vi "s-6 metin belgesindeki datayı dışarı aktaran, okunmasını sağlayan program 2018 19.vi"() -> ()   [LabVIEW 2014]
panel:
  out "String":string
  in  "Path":path
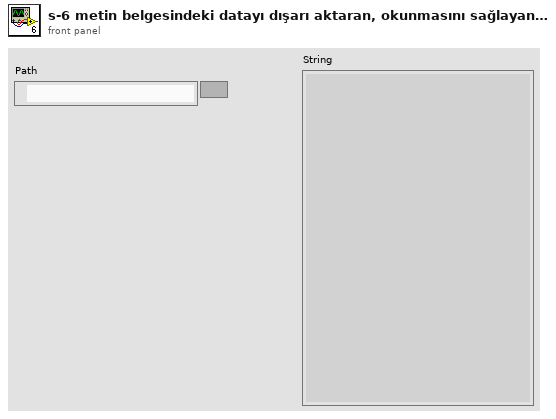
[diagram p1: front panel]
types:
  T1 = enum16{"open", "replace", "create", "open or create", "replace or create", "replace or create with confirmation"}
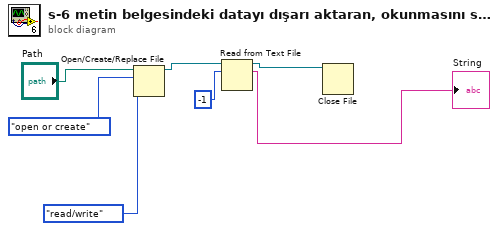
[diagram p0: block diagram]
diagram:
  n1 = Open/Create/Replace File(file path (use dialog)="Path", operation (0:open)=T1."open or create", access (0:read/write)=enum16{"read/write", "read-only", "write-only"}."read/write") -> (refnum out=w4:refnum<file>)  [unwired: 3 in, 2 out]
  n2 = Read from Text File(file (use dialog)=w4, count=-1) -> (refnum out=w2:refnum<file>, text=→"String":string)  [unwired: 2 in, 2 out]
  n3 = Close File(refnum=w2) -> ()  [unwired: 1 in, 2 out]
